vi "WFT AIO Configure.vi"(8 "Error In":errorcluster, 11 "WaveForms Session In":T1) -> (0 "Error Out":errorcluster, 2 "ret":i32, 3 "WaveForms Session Out":T1)   [LabVIEW 2020, in "lv_waveforms_toolkit.lvlib"]
uses:
  lv_waveforms_toolkit.lvlib
  WFT Session.ctl
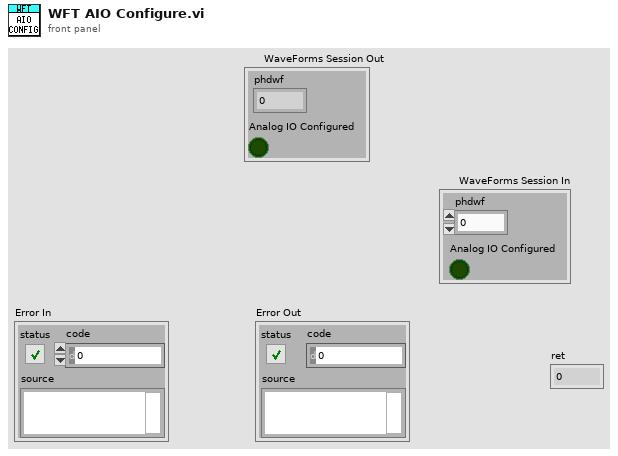
[diagram p1: front panel]
types:
  T1 = typedef "lv_waveforms_toolkit.lvlib/WFT Session.ctl" = cluster{"phdwf":i32, "Analog IO Configured":bool}
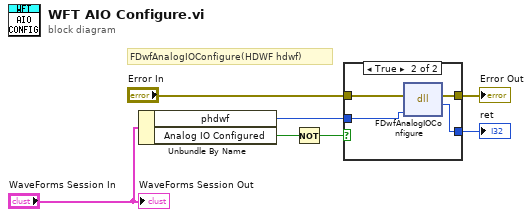
[diagram p0: block diagram]
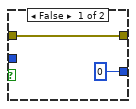
[diagram p2: hidden frame]
diagram:
  # "FDwfAnalogIOConfigure(HDWF hdwf)"
  n1 = Unbundle By Name("WaveForms Session In") -> ("phdwf"=w3:i32, "Analog IO Configured"=w2:bool)
  n2 = Not(x=w2) -> (.not. x?=w1:bool)
  n3 = case shown="True" w1 {
    tunnel: [0 ("return type") w13] -> w7
    tunnel: "Error In" -> [w9 w12]
    tunnel: [w9 w11] -> w5
    tunnel: w3 -> [_ w10]
    frame False {
    }
    frame True {
      n4 = dll-call lib="dwf" fn="FDwfAnalogIOConfigure"(error in=w12, "phdwf"=w10) -> (error out=w11:errorcluster, "return type"=w13:i32)  [unwired: 3 in, 1 out]
    }
  }
  "ret" <- w7
  "Error Out" <- w5
  "WaveForms Session Out" <- "WaveForms Session In"
